vi "断开市电.vi"   [LabVIEW 2016]
types:
  T1 = cluster{"命令":string, cluster{"starting address":u16, "holding register value":u16}}
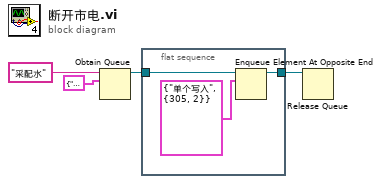
[diagram p0: block diagram]
diagram:
  n1 = Obtain Queue(name (unnamed)="采配水" ("名称（未命名）"), element data type=cluster{"命令":string, "数据":variant} {"命令"="", "数据"=variant}) -> (queue out=w2:refnum<queue>)  [unwired: 3 in, 2 out]
  n2 = flat-sequence {
    tunnel: w2 -> [w6]
    tunnel: [w5] -> w1
    frame #0 {
      n3 = Enqueue Element At Opposite End(queue=w6, element=T1 {"命令"="单个写入", {"starting address"=305, "holding register value"=2}} ("元素")) -> (queue out=w5:refnum<queue>)  [unwired: 2 in, 2 out]
    }
  }
  n4 = Release Queue(queue=w1) -> ()  [unwired: 2 in, 3 out]
